vi "_Get Control References[] from GObjects[].vi"(8 "error in":errorcluster, 11 "Objects[]":refnum<vi>[](array[refnum])) -> (0 "error out":errorcluster, 3 "Controls[]":refnum<vi>[](array[refnum]))   [LabVIEW 2012, in "Build Array of References__RCF.lvlib"]
doc: "Gets an array of references to controls from an array of Gobjects. If the Gobjects include local variables and terminals, gets the controls they are associated with as well."
uses:
  Build Array of References__RCF.lvlib
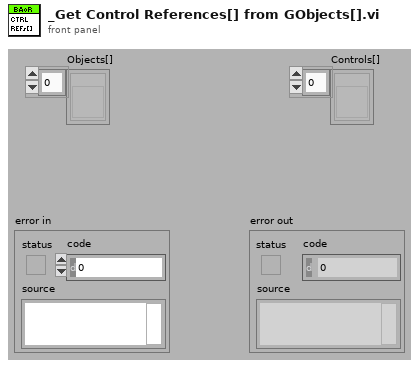
[diagram p1: front panel]
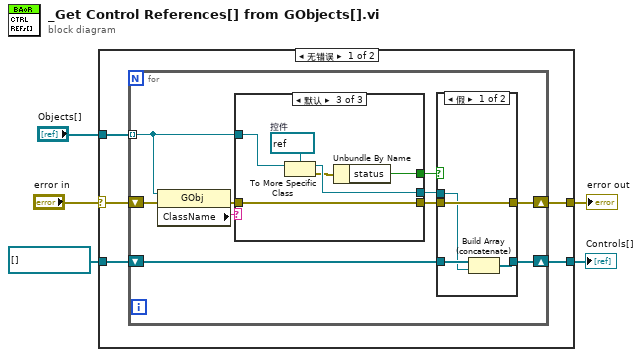
[diagram p0: block diagram]
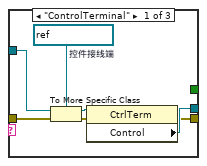
[diagram p3: hidden frame]
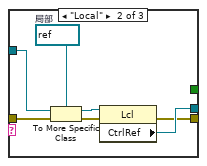
[diagram p4: hidden frame]
diagram:
  n1 = case shown="无错误" "error in" {
    selector: "error in" -> [w8 w47]
    tunnel: [w7 _] -> w5
    tunnel: [w6 w47] -> w4
    tunnel: "Objects[]" -> [w10 _]
    tunnel: refnum<vi>[] [] ("Array") -> [w9 _]
    frame No Error {
      n2 = for {
        tunnel: w10 -> [w19] mode=indexing
        shift-right: [w18] -> w7
        shift-left: w9 -> [w20]
        shift-right: [w17] -> w6
        shift-left: w8 -> [w16]
        n3 = property class="GObj"(reference=w19, error in=w16) -> (error out=w11:errorcluster, "ClassName"=w14:string)  [unwired: 1 out]
        n4 = case shown="默认" w14 {
          tunnel: w19 -> [w33 w40 w46]
          tunnel: [w29 w36 w44] -> w15
          tunnel: [w28 w35 w41] -> w12
          tunnel: [_ _ w42] -> w13
          tunnel: w11 -> [w27 w34 w41]
          frame "ControlTerminal" {
            w32 = refnum<vi> refnum  # 控件接线端
            n5 = To More Specific Class(target class=w32, reference=w33, error in=w27) -> (specific class reference=w31:refnum<vi>, error out=w30:errorcluster)
            n6 = property class="CtrlTerm"(reference=w31, error in=w30) -> (error out=w28:errorcluster, "Control"=w29:refnum<vi>)  [unwired: 1 out]
          }
          frame "Local" {
            w39 = refnum<vi> refnum  # 局部
            n7 = To More Specific Class(target class=w39, reference=w40, error in=w34) -> (specific class reference=w38:refnum<vi>, error out=w37:errorcluster)
            n8 = property class="Lcl"(reference=w38, error in=w37) -> (error out=w35:errorcluster, "CtrlRef"=w36:refnum<vi>)  [unwired: 1 out]
          }
          frame Default {
            w45 = refnum<vi> refnum  # 控件
            n9 = To More Specific Class(target class=w45, reference=w46) -> (specific class reference=w44:refnum<vi>, error out=w43:errorcluster)  [unwired: 1 in]
            n10 = Unbundle By Name(w43) -> ("status"=w42:bool)
          }
        }
        n11 = case shown="假" w13 {
          tunnel: w15 -> [w21 _]
          tunnel: w20 -> [w24 w26]
          tunnel: [w23 w26] -> w18
          tunnel: [w22 w25] -> w17
          tunnel: w12 -> [w22 w25]
          frame False {
            n12 = Build Array (concatenate)(w24, w21) -> (w23:refnum<vi>[])
          }
          frame True {
          }
        }
      }
    }
    frame Error {
    }
  }
  "Controls[]" <- w5
  "error out" <- w4
